vi "DrawImage.vi"(0 "reference in":refnum<class "LcPictureBox.lvclass">, 1 "UpperLeftCorner(0,0)":cluster{"x":sgl, "y":sgl}, 3 "Filename":path, 4 "Image":refnum<k24>, 5 "Error In":errorcluster, 7 "ScaleFactor(1)":sgl=1.0, 8 "SmoothingMode(AntiAlias)":T1=enum."AntiAlias", 9 "Rotation(Deg)":sgl) -> (14 "reference out":refnum<class "LcPictureBox.lvclass">, 15 "Graphics":refnum<k24>, 19 "Error Out":errorcluster)   [LabVIEW 2020, in "LcPictureBox.lvclass"]
uses:
  LcPictureBox.lvclass
  SmoothingMode.ctl
  System.Drawing
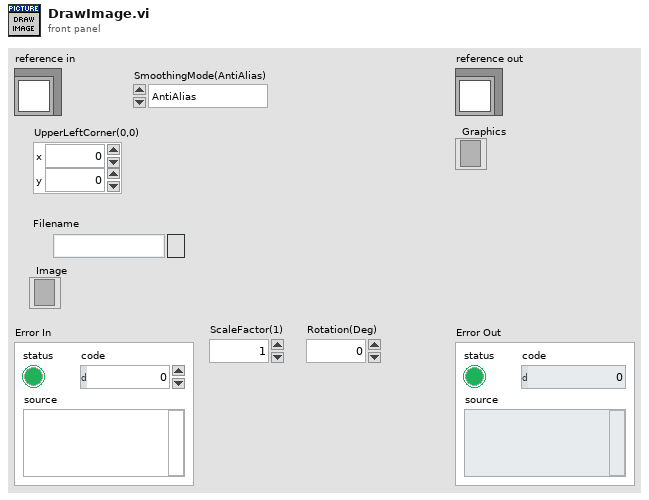
[diagram p1: front panel]
types:
  T1 = typedef "LcPictureBox.lvclass/SmoothingMode.ctl" = enum16{"None", "HighSpeed", "HighQuality", "AntiAlias"}
  T2 = typedef "LcPictureBox.lvclass/ObjectAttributes.ctl" = cluster{"PictureBox":refnum<k24>, "ImageSize":cluster{"Width":i32, "Height":i32}, "PenMemory":map{cluster{"Alpha(100%)":dbl, "Color(Black)":u32, "Pen(Width=1, Solid)":T3}, refnum<k24>}, "GraphicsRef":refnum<k24>, "BrushMemory":map{cluster{"Alpha(100%)":dbl, "Color(Black)":u32}, refnum<k24>}, "Images":refnum<k24>[], "ImageIndex":i32, "BgColor(None)":u32, "LoadedImages":map{string, cluster{"ImageOut":refnum<k24>, "ImageSize":cluster{"Width":i32, "Height":i32}}}, "ColorsMemory":map{cluster{"Alpha(100%)":dbl, "Color(Black)":u32}, refnum<k24>}, "CacheSize":i32, "PictureBoxActiveXReference":refnum<vi>, "Scale":dbl, "Offset":cluster{"x":sgl, "y":sgl}, "zoom_center":cluster{"X":i32, "Y":i32}, "ImagesCreated":refnum<k24>[], "CustomCursorImages":map{u16, refnum<k24>}}
  T3 = typedef "LcPictureBox.lvclass/Pen.ctl" = cluster{"Width":u16, "Style":enum32{"Solid", "Dash", "Dot", "DashDot", "DashDotDot"}}
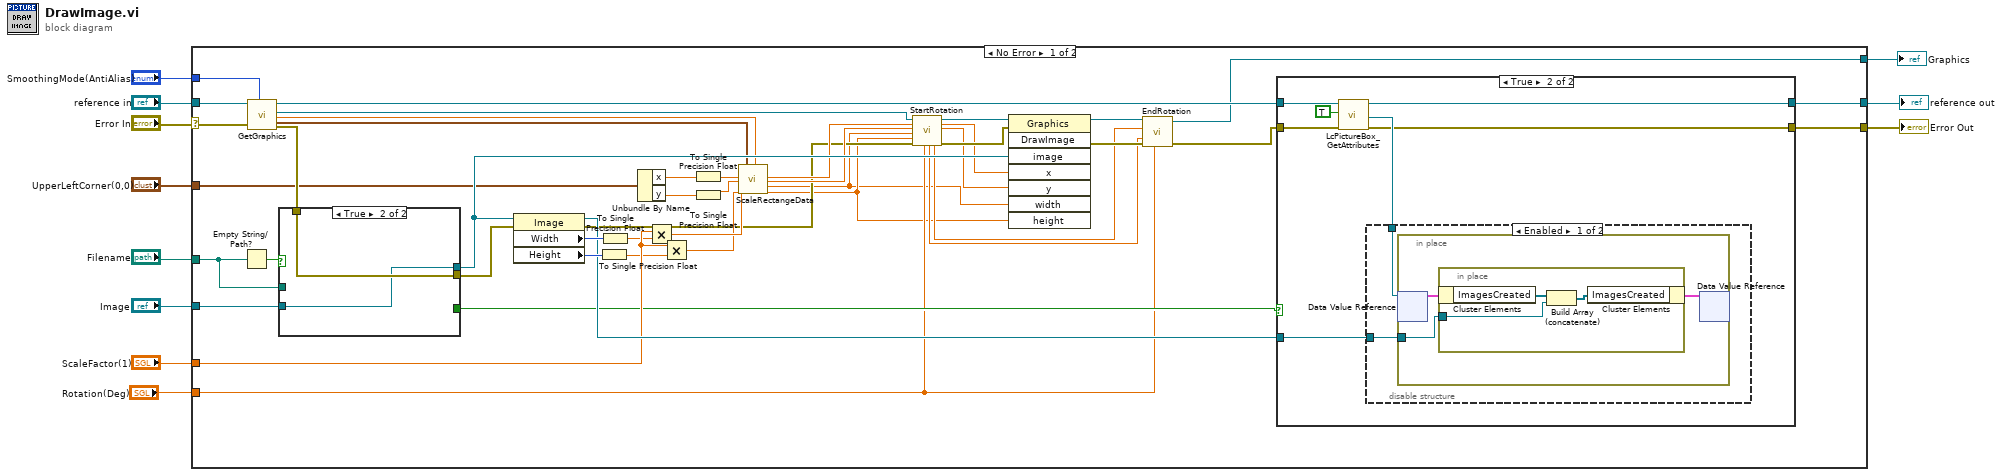
[diagram p0: block diagram]
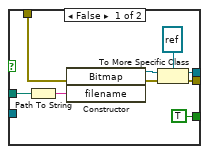
[diagram p2: hidden frame]
diagram:
  n1 = case shown="No Error" "Error In" {
    selector: "Error In" -> [w54 w86]
    tunnel: [w38 w86] -> w10
    tunnel: [w42 w85] -> w8
    tunnel: "reference in" -> [w52 w85]
    tunnel: "SmoothingMode(AntiAlias)" -> [w56 _]
    tunnel: "UpperLeftCorner(0,0)" -> [w45 _]
    tunnel: "Filename" -> [w51 _]
    tunnel: "Image" -> [w49 _]
    tunnel: "ScaleFactor(1)" -> [w37 _]
    tunnel: "Rotation(Deg)" -> [w16 _]
    tunnel: [w17 _] -> w1
    frame No Error {
      n2 = Empty String/Path?(string/path=w51) -> (empty?=w50:bool)
      n3 = call "GetGraphics.vi"("LcPictureBox in"=w52, "error in (no error)"=w54, "SmoothingMode"=w56) -> ("LcPictureBox out"=w43:refnum<class "LcPictureBox.lvclass">, "Graphics"=w28:refnum<k24>, "Scale"=w32:dbl, "Offset"=w31:cluster{"x":sgl, "y":sgl}, "error out"=w55:errorcluster)  [unwired: 12 in]
      n4 = case shown="True" w50 {
        tunnel: [w62 w66] -> w48
        tunnel: [w61 w67] -> w46
        tunnel: w55 -> [w60 w67]
        tunnel: w51 -> [w58 _]
        tunnel: w49 -> [_ w66]
        tunnel: [TRUE _] -> w36
        frame False {
          n5 = Path To String(path=w58) -> (string=w59:string)
          n6 = constructor class="Bitmap"(error in=w60, "filename"=w59) -> (reference out=w64:refnum<k24>, error out=w63:errorcluster)  [unwired: 2 in, 2 out]
          n7 = To More Specific Class(target class=refnum<k24> refnum, reference=w64, error in=w63) -> (specific class reference=w62:refnum<k24>, error out=w61:errorcluster)
        }
        frame True {
        }
      }
      n8 = property class="Image"(reference=w48, error in=w46) -> (reference out=w39:refnum<k24>, error out=w21:errorcluster, "Width"=w41:i32, "Height"=w40:i32)
      n9 = To Single Precision Float(number=w40) -> (single precision float=w29:sgl)
      n10 = To Single Precision Float(number=w41) -> (single precision float=w30:sgl)
      n11 = Unbundle By Name(w45) -> ("x"=w44:sgl, "y"=w53:sgl)
      n12 = Multiply(x=w37, y=w30) -> (x*y=w47:sgl)
      n13 = Multiply(x=w37, y=w29) -> (x*y=w33:sgl)
      n14 = To Single Precision Float(number=w44) -> (single precision float=w35:sgl)
      n15 = To Single Precision Float(number=w53) -> (single precision float=w34:sgl)
      n16 = call "ScaleRectangeData.vi"("X-In"=w35, "Y-In"=w34, "Width-In"=w47, "Height-In"=w33, "Offset(raw)"=w31, "Scale"=w32) -> ("X-Out"=w25:sgl, "Y-Out"=w23:sgl, "Width-Out"=w12:sgl, "Height-Out"=w13:sgl)  [unwired: 10 in]
      n17 = call "StartRotation.vi"("Graphics Refnum in"=w28, "X-In"=w25, "Y-In"=w23, "Width-In"=w12, "Height-In"=w13, "error in (no error)"=w21, "Rotation(Deg)"=w16) -> ("dyTranslation"=w15:sgl, "dxTranslation"=w14:sgl, "Graphics Refnum out"=w27:refnum<k24>, "X-Out"=w24:sgl, "Y-Out"=w22:sgl, "error out"=w26:errorcluster)  [unwired: 5 in, 2 out]
      n18 = invoke class="Graphics" method="DrawImage"(reference=w27, error in=w26, "image"=w48, "x"=w24, "y"=w22, "width"=w12, "height"=w13) -> (reference out=w20:refnum<k24>, error out=w19:errorcluster)  [unwired: 1 in, 6 out]
      n19 = call "EndRotation.vi"("Rotation(Deg)"=w16, "error in (no error)"=w19, "dyTranslation"=w15, "dxTranslation"=w14, ".NET Refnum in"=w20) -> ("error out"=w18:errorcluster, ".NET Refnum out"=w17:refnum<k24>)  [unwired: 5 in]
      n20 = case shown="True" w36 {
        tunnel: w43 -> [w69 w76]
        tunnel: [w69 w75] -> w42
        tunnel: w39 -> [_ w73]
        tunnel: w18 -> [w68 w72]
        tunnel: [w68 w71] -> w38
        frame False {
        }
        frame True {
          n21 = call "LcPictureBox_GetAttributes.vi"("reference in"=w76, "OnlyGetDvrReference(False)"=TRUE, "error in (no error)"=w72) -> ("reference out"=w75:refnum<class "LcPictureBox.lvclass">, "DataRef"=w74:refnum<data-value>, "error out"=w71:errorcluster)  [unwired: 13 in, 1 out]
          n22 = disable-structure shown="Enabled" {
            disable-tunnel: w74 -> [w78 _]
            disable-tunnel: w73 -> [w77 _]
            frame Enabled {
              n23 = in-place {
                in-place-border: w77 -> [w79]
                n24 = in-place-dvr #1(w78) -> (w81:T2)  [unwired: 1 out]
                n25 = in-place {
                  in-place-border: w79 -> [w84]
                  n26 = in-place-cluster #2(w81) -> ("ImagesCreated"=w83:refnum<k24>[])
                  n27 = Build Array (concatenate)(w83, w84) -> (w82:refnum<k24>[])
                  n28 = in-place-cluster #2("ImagesCreated"=w82) -> (w80:T2)
                }
                n29 = in-place-dvr #1(w80) -> ()  [unwired: 2 out]
              }
            }
            frame Disabled {
            }
          }
        }
      }
    }
    frame Error {
    }
  }
  "Error Out" <- w10
  "reference out" <- w8
  "Graphics" <- w1
